vi "DAQ create sandbox.vi"() -> ()   [LabVIEW 2016]
uses:
  <vilib>/DAQmx/create/channels.llb/DAQmx Create Channel (AI-Voltage-Basic).vi
  <vilib>/DAQmx/configure/timing.llb/DAQmx Timing (Sample Clock).vi
  <vilib>/DAQmx/configure/trigger.llb/DAQmx Start Trigger (Digital Edge).vi
  <resource>/objmgr/daqmx.rc
panel:
  in  "buffer size (in samples per channel)":u32
  in  "rate":dbl=1000.0 format="%0.2f"
  in  "AI.Channels":string
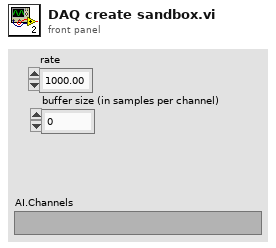
[diagram p1: front panel]
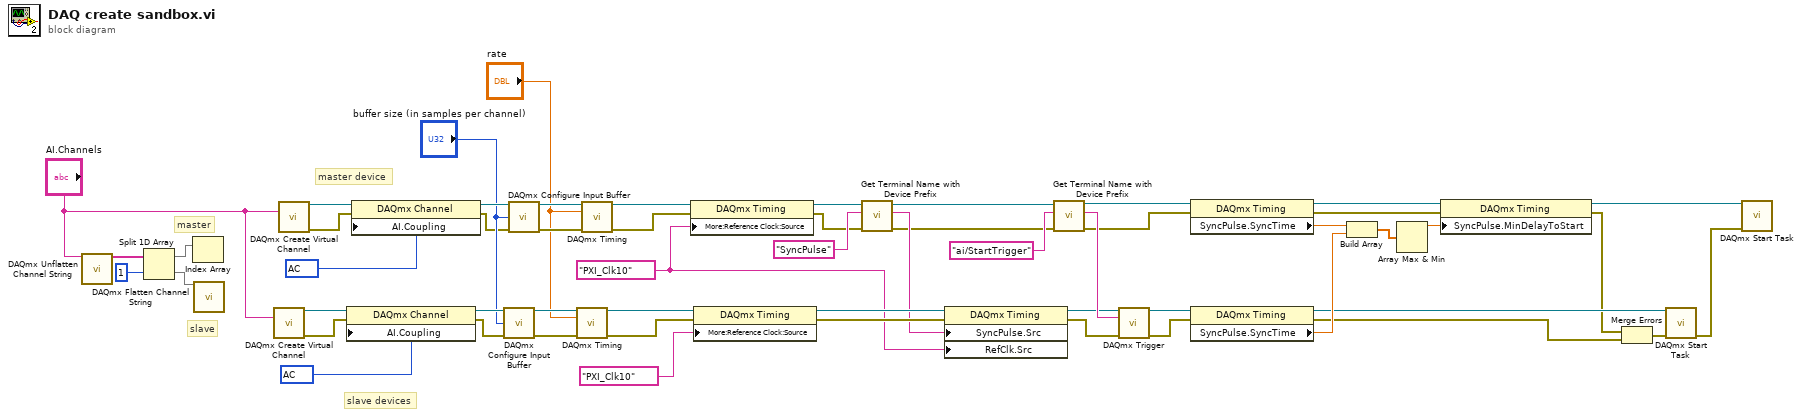
[diagram p0: block diagram]
diagram:
  w38 = 10045 items=["AC"=10045, "DC"=10050, "GND"=10066] ("AI.Coupling")
  w32 = tag "PXI_Clk10" ("RefClk.Src")
  w53 = 10045 items=["AC"=10045, "DC"=10050, "GND"=10066] ("AI.Coupling")
  # "slave"
  # "master"
  # "slave devices"
  # "master device"
  n1 = call <vilib>:"DAQmx Unflatten Channel String.vi"("names in"="AI.Channels") -> ("names out"=w4:string[])  [unwired: 13 in, 1 out]
  n2 = Split 1D Array(array=w4, index=1 ("length")) -> (first subarray=w3:string[], second subarray=w2:string[])
  n3 = Index Array(array=w3) -> ()  [unwired: 1 in, 1 out]
  n4 = call <vilib>:"DAQmx Flatten Channel String.vi"("names in"=w2) -> ()  [unwired: 13 in, 2 out]
  n5 = call-poly <vilib>:"DAQmx Create Virtual Channel.vi"("physical channels"="AI.Channels") -> ("task out"=w36:refnum<k21>, "error out"=w37:errorcluster)  [unwired: 13 in]
  n6 = call-poly <vilib>:"DAQmx Create Virtual Channel.vi"("physical channels"="AI.Channels") -> ("task out"=w55:refnum<k21>, "error out"=w54:errorcluster)  [unwired: 13 in]
  n7 = property class="DAQmx Channel"(reference=w36, error in=w37, "AI.Coupling"=w38) -> (reference out=w39:refnum<k21>, error out=w29:errorcluster)
  n8 = property class="DAQmx Channel"(reference=w55, error in=w54, "AI.Coupling"=w53) -> (reference out=w52:refnum<k21>, error out=w28:errorcluster)
  n9 = call <vilib>:"DAQmx Configure Input Buffer.vi"("task/channels in"=w39, "buffer size (in samples per channel)"="buffer size (in samples per channel)", "error in"=w29) -> ("task out"=w40:refnum<k21>, "error out"=w41:errorcluster)  [unwired: 11 in]
  n10 = call <vilib>:"DAQmx Configure Input Buffer.vi"("task/channels in"=w52, "buffer size (in samples per channel)"="buffer size (in samples per channel)", "error in"=w28) -> ("task out"=w51:refnum<k21>, "error out"=w50:errorcluster)  [unwired: 11 in]
  n11 = call-poly <vilib>:"DAQmx Timing.vi"("task/channels in"=w40, "rate"="rate", "error in"=w41) -> ("task out"=w44:refnum<k21>, "error out"=w42:errorcluster)  [unwired: 11 in]
  n12 = call-poly <vilib>:"DAQmx Timing.vi"("task/channels in"=w51, "rate"="rate", "error in"=w50) -> ("task out"=w48:refnum<k21>, "error out"=w49:errorcluster)  [unwired: 11 in]
  n13 = property class="DAQmx Timing"(reference=w48, error in=w49, "More:Reference Clock:Source"=w32) -> (reference out=w47:refnum<k21>, error out=w45:errorcluster)
  n14 = property class="DAQmx Timing"(reference=w44, error in=w42, "More:Reference Clock:Source"=tag "PXI_Clk10" ("RefClk.Src")) -> (reference out=w35:refnum<k21>, error out=w34:errorcluster)
  n15 = call "Get Terminal Name with Device Prefix.vi"("error in (no error)"=w45, "Local Terminal Name"="SyncPulse", "task/channels in"=w47) -> ("error out"=w26:errorcluster, "Terminal Name with Device Prefix"=w33:tag, "task out"=w25:refnum<k21>)  [unwired: 6 in]
  n16 = property class="DAQmx Timing"(reference=w35, error in=w34, "SyncPulse.Src"=w33, "RefClk.Src"=w32) -> (reference out=w23:refnum<k21>, error out=w22:errorcluster)
  n17 = call "Get Terminal Name with Device Prefix.vi"("error in (no error)"=w26, "Local Terminal Name"="ai/StartTrigger", "task/channels in"=w25) -> ("error out"=w15:errorcluster, "Terminal Name with Device Prefix"=w24:tag, "task out"=w16:refnum<k21>)  [unwired: 6 in]
  n18 = call-poly <vilib>:"DAQmx Trigger.vi"("task/channels in"=w23, "source"=w24, "error in"=w22) -> ("task out"=w14:refnum<k21>, "error out"=w13:errorcluster)  [unwired: 11 in]
  n19 = property class="DAQmx Timing"(reference=w16, error in=w15) -> (reference out=w19:refnum<k21>, error out=w20:errorcluster, "SyncPulse.SyncTime"=w21:dbl)
  n20 = property class="DAQmx Timing"(reference=w14, error in=w13) -> (reference out=w9:refnum<k21>, error out=w6:errorcluster, "SyncPulse.SyncTime"=w12:dbl)
  n21 = Build Array(w21, w12) -> (w18:dbl[])
  n22 = Array Max & Min(array=w18) -> (max value=w17:dbl)  [unwired: 3 out]
  n23 = property class="DAQmx Timing"(reference=w19, error in=w20, "SyncPulse.MinDelayToStart"=w17) -> (reference out=w11:refnum<k21>, error out=w7:errorcluster)
  n24 = Merge Errors(w7, w6) -> (w8:errorcluster)
  n25 = call <vilib>:"DAQmx Start Task.vi"("task/channels in"=w9, "error in"=w8) -> ("error out"=w10:errorcluster)  [unwired: 12 in, 1 out]
  n26 = call <vilib>:"DAQmx Start Task.vi"("task/channels in"=w11, "error in"=w10) -> ()  [unwired: 12 in, 2 out]
